vi "IO@Flash(OffOn)__Parameter.vi"(1 "ParamterIn":string) -> (0 "ParamterOut":string)   [LabVIEW 2020]
panel:
  in  "Delay On":string(combo)
  in  "Delay off":string(combo)
  in  "PortSelect":string(combo)
  in  "Confirm":bool
  # "IO@Flash(OnOff)/(OffOn) $IOName,$On Delay(,$Off Delay )"
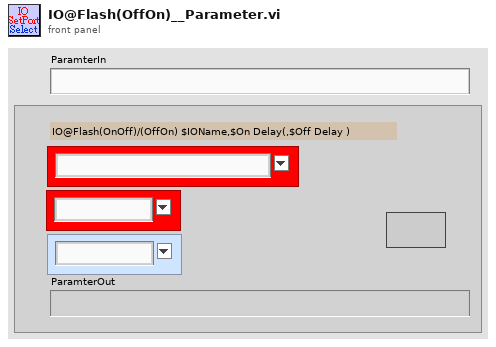
[diagram p1: front panel]
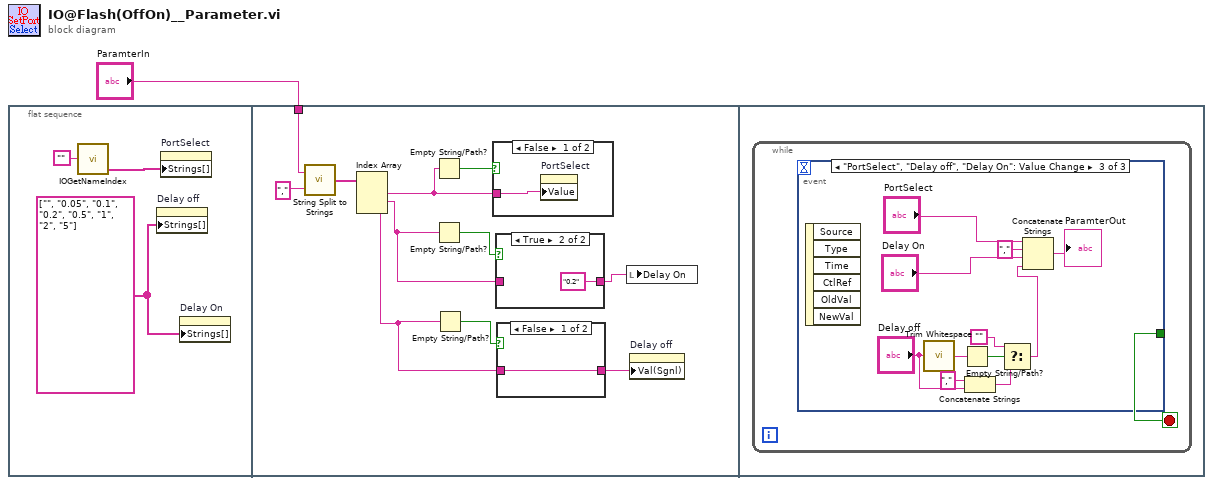
[diagram p0: block diagram]
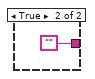
[diagram p2: hidden frame]
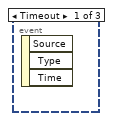
[diagram p5: hidden frame]
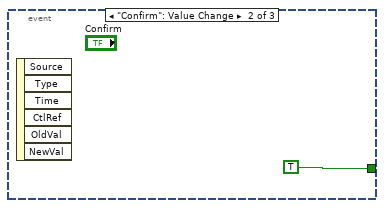
[diagram p6: hidden frame]
diagram:
  n1 = flat-sequence {
    tunnel: "ParamterIn" -> [w13]
    frame #0 {
      w2 = string[] ["", "0.05", "0.1", "0.2", "0.5", "1", "2", "5"] ("Strings []")
      n2 = call "IOGetNameIndex.vi"("PortName"="") -> ("PortNameList Out"=w3:string[])  [unwired: 3 in, 1 out]
      n3 = property on="Delay off" class="CmbBox"("Strings[]"=w2) -> ()  [unwired: 2 in, 2 out]
      n4 = property on="PortSelect" class="CmbBox"("Strings[]"=w3) -> ()  [unwired: 2 in, 2 out]
      n5 = property on="Delay On" class="CmbBox"("Strings[]"=w2) -> ()  [unwired: 2 in, 2 out]
    }
    frame #1 {
      n6 = call "String Split to Strings.vi"("search string/char (-)"=",", "String"=w13) -> ("Array"=w14:string[])
      n7 = Index Array(array=w14) -> (element #1=w11:string, element #2=w9:string, element #3=w7:string)  [unwired: 3 in]
      n8 = Empty String/Path?(string/path=w11) -> (empty?=w12:bool)
      n9 = Empty String/Path?(string/path=w9) -> (empty?=w10:bool)
      n10 = Empty String/Path?(string/path=w7) -> (empty?=w8:bool)
      n11 = case shown="False" w12 {
        tunnel: w11 -> [w20 _]
        frame False {
          n12 = property on="PortSelect" class="CmbBox"("Value"=w20) -> ()  [unwired: 2 in, 2 out]
        }
        frame True {
        }
      }
      n13 = case shown="True" w10 {
        tunnel: [w18 "0.2"] -> w5
        tunnel: w9 -> [w18 _]
        frame False {
        }
        frame True {
        }
      }
      n14 = case shown="False" w8 {
        tunnel: [w16 ""] -> w6
        tunnel: w7 -> [w16 _]
        frame False {
        }
        frame True {
        }
      }
      n15 = local write "Delay On"(w5) -> ()
      n16 = property on="Delay off" class="CmbBox"("Val(Sgnl)"=w6) -> ()  [unwired: 2 in, 2 out]
    }
    frame #2 {
      n17 = while {
        stop <- w21 stop-if-true
        n18 = event shown="[2] \"PortSelect\", \"Delay off\", \"Delay On\": Value Change" {
          selector: _ -> [_ _ _]
          dyn-events: _ -> [_ _ _]
          timeout: _ -> [_ _ _]
          tunnel: [_ TRUE _] -> w21
          event Timeout {
            n19 = event-data() -> ()  [unwired: 1 in, 3 out]
          }
          event "Confirm": Value Change {
            n20 = event-data() -> ()  [unwired: 1 in, 6 out]
          }
          event "PortSelect", "Delay off", "Delay On": Value Change {
            n21 = event-data() -> ()  [unwired: 1 in, 6 out]
            n22 = call <vilib>:"Trim Whitespace.vi"("string"="Delay off") -> ("trimmed string"=w31:string)  [unwired: 1 in]
            n23 = Empty String/Path?(string/path=w31) -> (empty?=w30:bool)
            n24 = Concatenate Strings("," ("string"), "Delay off") -> (w28:string)
            n25 = Select(t="", s=w30, f=w28) -> (s? t:f=w25:string)
            n26 = Concatenate Strings("PortSelect", "," ("string"), "Delay On", w25) -> (→"ParamterOut":string)
          }
        }
      }
    }
  }
